vi "PQsetClientEncoding.vi"(9 "encode":string, 11 "conn":u32) -> (1 "PQsetClientEncoding":i32, 3 "conn_out":u32)   [LabVIEW 2019, in "libpqutility64.lvlib"]
doc: "Character Set Encoding for Client.\nFor further Information see PostgreSQL c-lib documentation"
uses:
  libpqutility64.lvlib
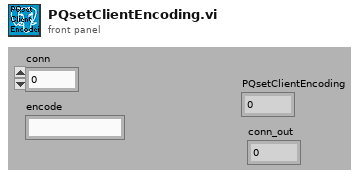
[diagram p1: front panel]
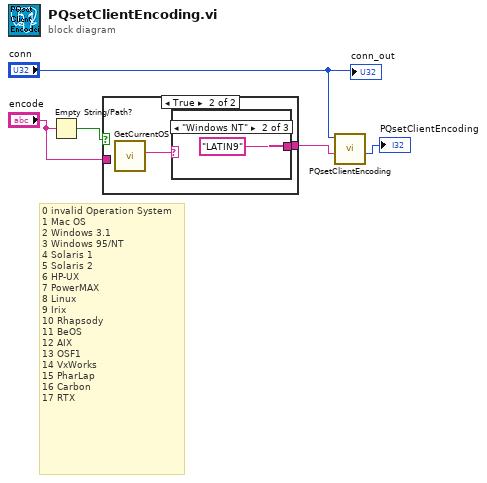
[diagram p0: block diagram]
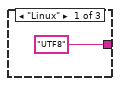
[diagram p3: hidden frame]
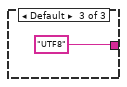
[diagram p4: hidden frame]
diagram:
  # "0 invalid Operation System\n1 Mac OS \n2 Windows 3.1 \n3 Windows 95/NT \n4 Solaris 1 \n5 Solaris 2 \n6 HP-UX \n7 PowerMAX \n8 Linux \n9 Irix \n10 Rhapsody \n11 BeOS \n12 AIX \n13 OSF1 \n14 VxWorks \n15 PharLap \n16 Carbon \n17 RTX"
  n1 = Empty String/Path?(string/path="encode") -> (empty?=w4:bool)
  n2 = case shown="True" w4 {
    tunnel: [w6 w8] -> w2
    tunnel: "encode" -> [w6 _]
    frame False {
    }
    frame True {
      n3 = call "GetCurrentOS.vi"() -> ("Betriebssystem:Name"=w7:string)  [unwired: 11 in]
      n4 = case shown="\"Windows NT\"" w7 {
        tunnel: ["UTF8" ("encoding") "LATIN9" ("encoding") "UTF8" ("encoding")] -> w8
        frame "Linux" {
        }
        frame "Windows NT" {
        }
        frame Default {
        }
      }
    }
  }
  n5 = call "PQsetClientEncoding.vi"("encode"=w2, "conn"="conn") -> ("PQsetClientEncoding"=→"PQsetClientEncoding":i32)  [unwired: 8 in, 1 out]
  "conn_out" <- "conn"
